vi "DCC Set Single Parameter.vi"(6 "Parameter IDs":T1, 7 "New Value":sgl, 8 "Error In":errorcluster, 10 "Module No":i16, 11 "DLL Path":path) -> (0 "Error Out":errorcluster, 2 "Module No":i16, 3 "DLL Path":path)   [LabVIEW 2019]
doc: "The procedure sends the choose parameter with its new value to the internal DLL structures to the control registers of the DCC module specified by module number.\n\nThe new parameter value is recalculated according to the parameter limits and hardware restrictions. Furthermore, cross dependencies between different parameters are taken into account to ensure the correct hardware operation. It is recommended to read back the parameters after setting to get their true values after recalculation.\nThe values of ‘base_adr’ and ‘active’ are not changed. They can be changed only by a new ini_file an a DCC_init call. If an error occurs for a particular parameter it returns san error code. \n\nAugust 2018\nFrank Quadt & Stefan Smietana\ninfo@becker-hickl.com"
uses:
  DCC_Controls/DCC_ParameterIDs.ctl
panel:
  # "(c) 2021 Becker & Hickl GmbH\n     All Rights Reserved."
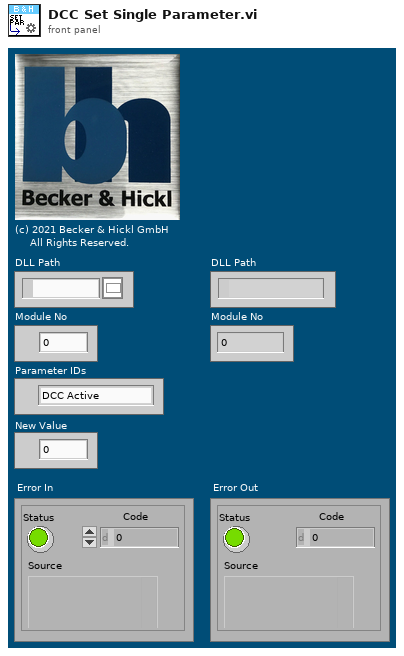
[diagram p1: front panel]
types:
  T1 = typedef "DCC_ParameterIDs.ctl" = enum16{"DCC Active", "PCI BUS No", "C1 +5 V", "C1-5 V", "C1 +12 V", "C1 Gain HV[%]", "C2 +5 V", "C2 -5 V", "C2 +12 V", "C2 Digout", "C3 Cooling", "C3 Cooling [V]", "C3 Cooling [A]", "C3 Gain HV [%]", "C3 +5 V", "C3 -5 V", "C3 +12 V"}
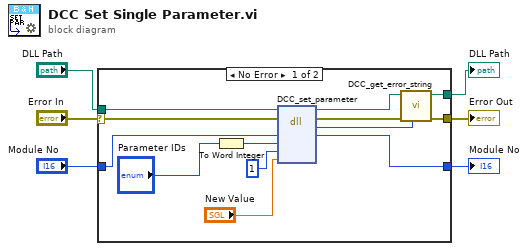
[diagram p0: block diagram]
diagram:
  n1 = case shown="No Error" "Error In" {
    selector: "Error In" -> [w19 w21]
    tunnel: [w15 w21] -> w5
    tunnel: [w14 w20] -> w4
    tunnel: "DLL Path" -> [w18 w20]
    tunnel: "Module No" -> [w13 w22]
    tunnel: [w11 w22] -> w1
    frame No Error {
      n2 = To Word Integer(number="Parameter IDs") -> (16bit integer=w7:i16)
      n3 = dll-call lib="C:/Program Files (x86)/BH/DCC/DLL/dcc64.dll" fn="DCC_set_parameter"(path in=w18, error in=w19, "ModuleNo"=w13, "ParameterID"=w7, "Send2Hard"=i16 1, "NewValue"="New Value") -> (path out=w17:path, error out=w16:errorcluster, "return type"=w12:i16, "ModuleNo"=w11:i16)  [unwired: 4 in]
      n4 = call "DCC_get_error_string.vi"("Error ID"=w12, "Error In"=w16, "DLL Path"=w17) -> ("Error Out"=w15:errorcluster, "DLL Path"=w14:path)  [unwired: 6 in, 1 out]
    }
    frame Error {
    }
  }
  "Error Out" <- w5
  "DLL Path" <- w4
  "Module No" <- w1
